vi "FT_Get_Device_Info.vi"(0 "Handle":u32, 11 "Error In":errorcluster) -> (4 "FT_Status":u32(ring) items=["FT_OK", "FT_INVALID_HANDLE", "FT_DEVICE_NOT_FOUND", "FT_DEVICE_NOT_OPENED", "FT_IO_ERROR", "FT_INSUFFICIENT_RESOURCES", "FT_INVALID_PARAMETER", "FT_INVALID_BAUD_RATE", "FT_DEVICE_NOT_OPENED_FOR_ERASE", "FT_DEVICE_NOT_OPENED_FOR_WRITE", "FT_FAILED_TO_WRITE_DEVICE", "FT_EEPROM_READ_FAILED", "FT_EEPROM_WRITE_FAILED", "FT_EEPROM_ERASE_FAILED", "FT_EEPROM_NOT_PRESENT", "FT_EEPROM_NOT_PROGRAMMED", "FT_INVALID_ARGS", "FT_NOT_SUPPORTED", "FT_OTHER_ERROR"], 6 "Device Information":T1 {"Type" items=["FT232B-FT245B", "FT8U232AM-FT8U245AM", "FT8U100AX", "UNKNOWN", "FT2232", "FT232R-FT245R", "FT2232H", "FT4232H", "FT232H"]}, 15 "Error Out":errorcluster)   [LabVIEW 2020]
uses:
  GEA3 DLL Source/ftd2xx.dll
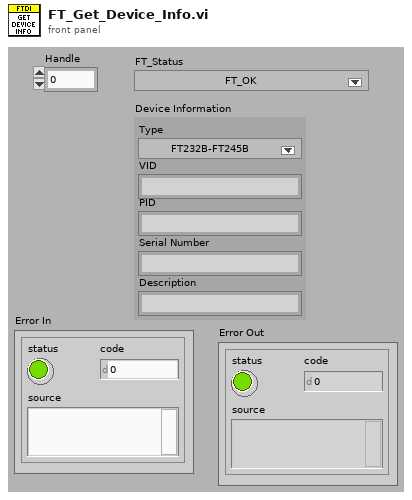
[diagram p1: front panel]
types:
  T1 = cluster{"Type":u32, "VID":string, "PID":string, "Serial Number":string, "Description":string}
  T2 = cluster{"DeviceType":u32, string, string, "SerialNumber":string, "Description":string}
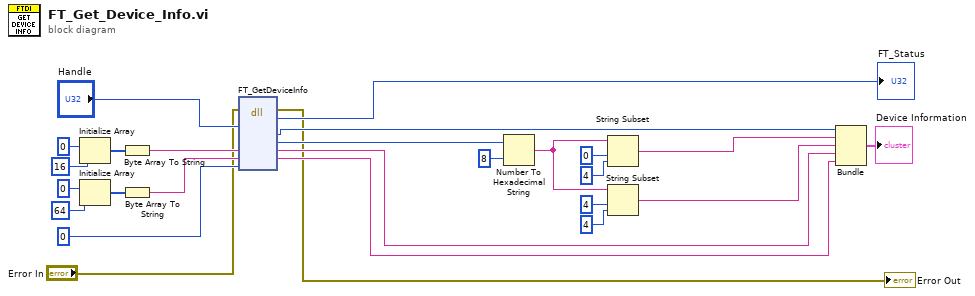
[diagram p0: block diagram]
diagram:
  n1 = Initialize Array(u8 0, 16 ("dimension size")) -> (w10:u8[])
  n2 = Initialize Array(u8 0, 64 ("dimension size")) -> (w8:u8[])
  n3 = Byte Array To String(unsigned byte array=w10) -> (string=w4:string)
  n4 = Byte Array To String(unsigned byte array=w8) -> (string=w5:string)
  n5 = dll-call lib="C:/TechnologyLab/NI-2010/Drivers/GEA3 Toolkit/GEA3 DLL Source/FTD2XX.dll" fn="FT_GetDeviceInfo"(error in="Error In", "Handle"="Handle", "SerialNumber"=w4, "Description"=w5, "Dummy"=u32 0) -> (error out=→"Error Out":errorcluster, "FT_Status"=→"FT_Status":u32, "DeviceType"=w3:u32, "ID"=w24:u32, "SerialNumber"=w15:string, "Description"=w14:string)  [unwired: 6 in, 1 out]
  n6 = Number To Hexadecimal String(1:i16 8 ("width (-)"), 2:w24) -> (0:w18:string)
  n7 = String Subset(string=w18, offset (0)=0, length (rest)=4 ("length (rest)")) -> (substring=w17:string)
  n8 = String Subset(string=w18, offset (0)=4, length (rest)=4 ("length (rest)")) -> (substring=w16:string)
  n9 = Bundle("DeviceType"=w3, w17, w16, "SerialNumber"=w15, "Description"=w14) -> (→"Device Information":T2)  [unwired: 1 in]
